vi "build.vi"(8 "error in (no error)":errorcluster, 11 "U8ArrayBuilderManualIndexing in":refnum<class "U8ArrayBuilderManualIndexing.lvclass">) -> (0 "error out":errorcluster, 2 "Array":u8[](array[numeric]), 3 "U8ArrayBuilderManualIndexing out":refnum<class "U8ArrayBuilderManualIndexing.lvclass">)   [LabVIEW 2016, in "RTUtilities.lvlib" / "U8ArrayBuilderManualIndexing.lvclass"]
uses:
  U8ArrayBuilderManualIndexing.lvclass
  U8ArrayBuilderManualIndexing.lvclass/U8ArrayBuilderManualIndexing.ctl
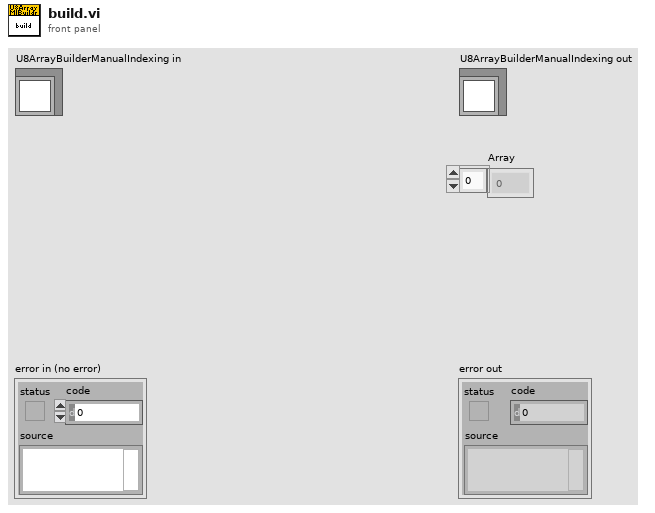
[diagram p1: front panel]
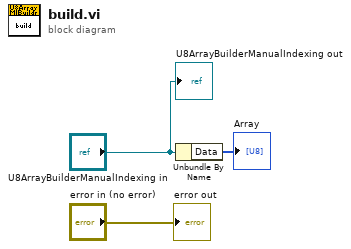
[diagram p0: block diagram]
diagram:
  n1 = Unbundle By Name("U8ArrayBuilderManualIndexing in") -> ("Data"=→"Array":u8[])
  "error out" <- "error in (no error)"
  "U8ArrayBuilderManualIndexing out" <- "U8ArrayBuilderManualIndexing in"
